vi "Get_Data_INI.vi"(0 "Application_Directory":path, 2 "Section":string, 5 "File_Name":path, 11 "Error_In":errorcluster, 13 "Key":string) -> (4 "Data":string, 15 "Error_Out":errorcluster)   [LabVIEW 2023]
uses:
  <vilib>/Utility/config.llb/Read Key (String).vi
  <vilib>/Utility/config.llb/NI_LVConfig.lvlib
panel:
  out "File_Path_Out":path
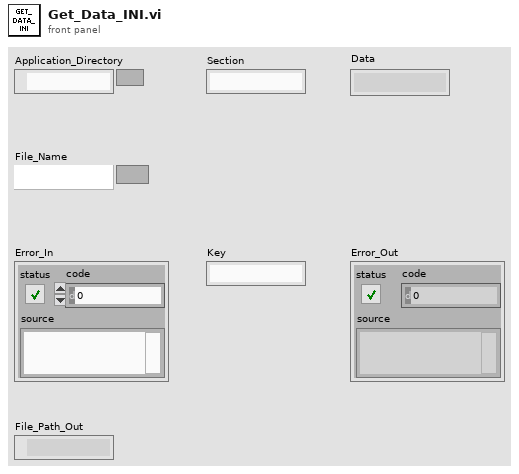
[diagram p1: front panel]
types:
  T1 = typedef "NI_LVConfig.lvlib/Config Data RefNum.ctl" = refnum<k1>
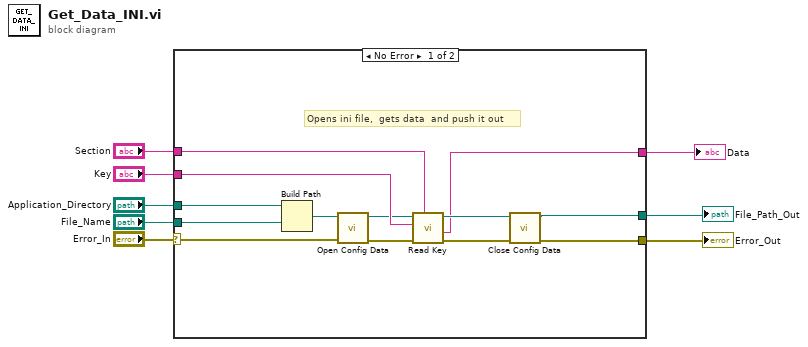
[diagram p0: block diagram]
diagram:
  n1 = case shown="No Error" "Error_In" {
    selector: "Error_In" -> [w12 w23]
    tunnel: "Application_Directory" -> [w19 w22]
    tunnel: "Key" -> [w17 _]
    tunnel: "Section" -> [w16 _]
    tunnel: [w13 _] -> w5
    tunnel: [w11 w23] -> w3
    tunnel: [w10 w22] -> w2
    tunnel: "File_Name" -> [w9 _]
    frame No Error {
      # "Opens ini file,  gets data  and push it out"
      n2 = Build Path(base path=w19, name or relative path=w9) -> (appended path=w18:path)
      n3 = call <vilib>:"Open Config Data.vi"("error in (no error)"=w12, "configuration file path"=w18) -> ("error out"=w21:errorcluster, "refnum"=w14:T1)  [unwired: 7 in, 1 out]
      n4 = call-poly <vilib>:"Read Key.vi"("section"=w16, "error in (no error)"=w21, "key"=w17, "refnum"=w14) -> ("error out"=w20:errorcluster, "value"=w13:string, "refnum out"=w15:T1)  [unwired: 4 in, 1 out]
      n5 = call <vilib>:"Close Config Data.vi"("error in (no error)"=w20, "refnum"=w15) -> ("error out"=w11:errorcluster, "file path"=w10:path)  [unwired: 8 in]
    }
    frame Error {
    }
  }
  "Data" <- w5
  "Error_Out" <- w3
  "File_Path_Out" <- w2
